vi "GetAllGtags.vi"(0 "tag":string, 1 "sdf in":string) -> (2 "Parameters":cluster{"key":string, "value":string}[][](array[cluster]), 3 "contents":string[](array[string]), 4 "sdf left":string)   [LabVIEW 2010]
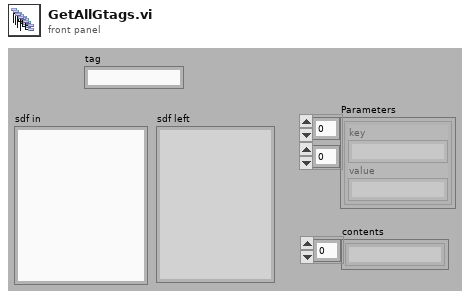
[diagram p1: front panel]
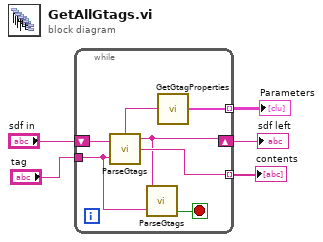
[diagram p0: block diagram]
diagram:
  n1 = while {
    tunnel: "tag" -> [w9]
    shift-right: [w10] -> w5
    shift-left: "sdf in" -> [w12]
    tunnel: [w11] -> w4 mode=indexing
    tunnel: [w6] -> w1 mode=indexing
    stop <- w8 stop-if-true
    n2 = call "ParseGtags.vi"("tag"=w9, "urdf in"=w12) -> ("parameters"=w7:string, "contents"=w11:string, "urdf out"=w10:string)  [unwired: 1 out]
    n3 = call "ParseGtags.vi"("tag"=w9, "urdf in"=w10) -> ("not found"=w8:bool)  [unwired: 3 out]
    n4 = call "GetGtagProperties.vi"("parameters"=w7) -> ("Parameters"=w6:cluster{"key":string, "value":string}[])
  }
  "sdf left" <- w5
  "contents" <- w4
  "Parameters" <- w1
